vi "Find Object Layout Index by Unique Name.vi"(8 "error in":errorcluster, 9 "unique name":string, 10 "object ID list in":variant, 11 "object layouts in":refnum<class "Object Layout.lvclass">[](array[class])) -> (0 "error out":errorcluster, 1 "found?":bool, 2 "object ID list out":variant, 3 "object layouts out":refnum<class "Object Layout.lvclass">[](array[class]), 5 "object layout index":i32)   [LabVIEW 2010, in "NI_SE_Front Panel Layout.lvlib"]
uses:
  NI_SE_Front Panel Layout.lvlib
  Object Layout Classes/Object Layout/Object Layout.lvclass
  Object Layout Classes/Object Layout/Object Layout.lvclass/Object Layout.ctl
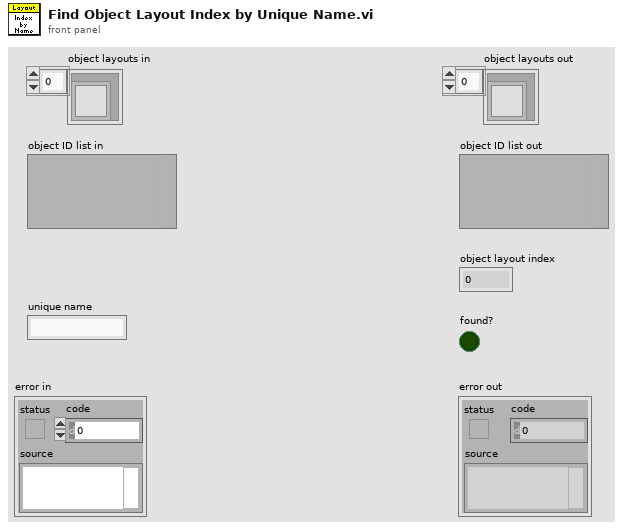
[diagram p1: front panel]
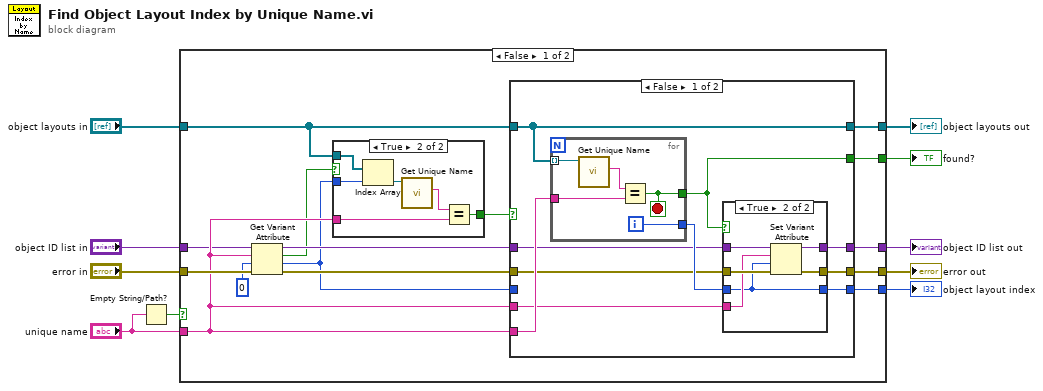
[diagram p0: block diagram]
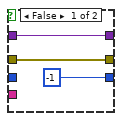
[diagram p3: hidden frame]
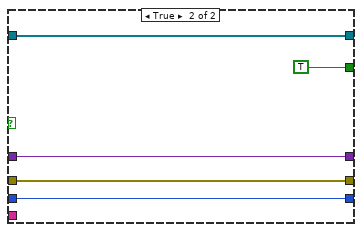
[diagram p4: hidden frame]
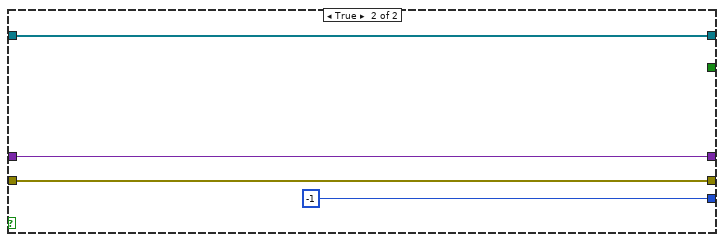
[diagram p5: hidden frame]
diagram:
  n1 = Empty String/Path?(string/path="unique name") -> (empty?=w2:bool)
  n2 = case shown="False" w2 {
    tunnel: "error in" -> [w25 w64]
    tunnel: [w24 w64] -> w6
    tunnel: [w23 -1] -> w8
    tunnel: [w22 _] -> w7
    tunnel: "unique name" -> [w21 _]
    tunnel: "object layouts in" -> [w20 w61]
    tunnel: "object ID list in" -> [w19 w62]
    tunnel: [w18 w62] -> w3
    tunnel: [w11 w61] -> w1
    frame False {
      n3 = Get Variant Attribute(Variant=w19, name=w21, default value (empty Variant)=0, error in=w25) -> (duplicate Variant=w16:variant, found=w13:bool, value=w14:i32, error out=w15:errorcluster)
      n4 = case shown="True" w13 {
        tunnel: w20 -> [_ w31]
        tunnel: w14 -> [_ w30]
        tunnel: w21 -> [_ w27]
        tunnel: [_ w26] -> w12
        frame False {
        }
        frame True {
          n5 = Index Array(array=w31, index=w30) -> (element=w29:refnum<class "Object Layout.lvclass">)
          n6 = call "Get Unique Name.vi"("Object Layout in"=w29) -> ("unique name"=w28:string)  [unwired: 7 in, 3 out]
          n7 = Equal?(x=w28, y=w27) -> (x = y?=w26:bool)
        }
      }
      n8 = case shown="False" w12 {
        tunnel: w20 -> [w32 w56]
        tunnel: w16 -> [w36 w60]
        tunnel: [w35 w60] -> w18
        tunnel: w14 -> [_ w57]
        tunnel: w15 -> [w33 w59]
        tunnel: [w39 w59] -> w24
        tunnel: [w40 w57] -> w23
        tunnel: [w34 TRUE] -> w22
        tunnel: w21 -> [w41 _]
        tunnel: w21 -> [w38 _]
        tunnel: [w32 w56] -> w11
        frame False {
          n9 = for {
            tunnel: w32 -> [w55] mode=indexing
            tunnel: [w54] -> w34
            tunnel: w41 -> [w53]
            tunnel: [w51] -> w37
            i -> [w51]
            stop <- w54 stop-if-true
            n10 = call "Get Unique Name.vi"("Object Layout in"=w55) -> ("unique name"=w52:string)  [unwired: 7 in, 3 out]
            n11 = Equal?(x=w52, y=w53) -> (x = y?=w54:bool)
          }
          n12 = case shown="True" w34 {
            tunnel: [-1 w45] -> w40
            tunnel: [w43 w50] -> w39
            tunnel: w33 -> [w43 w49]
            tunnel: w36 -> [w44 w48]
            tunnel: w38 -> [_ w47]
            tunnel: w37 -> [_ w45]
            tunnel: [w44 w46] -> w35
            frame False {
            }
            frame True {
              n13 = Set Variant Attribute(Variant=w48, name=w47, value=w45, error in=w49) -> (Variant out=w46:variant, error out=w50:errorcluster)  [unwired: 1 out]
            }
          }
        }
        frame True {
        }
      }
    }
    frame True {
    }
  }
  "error out" <- w6
  "object layout index" <- w8
  "found?" <- w7
  "object ID list out" <- w3
  "object layouts out" <- w1
